vi "MergeFilesCreateFileHeader.vi"(4 "Error In":errorcluster, 7 "MergeFileConfig":T1) -> (0 "Error Out":errorcluster, 3 "TextFileHeader":string)   [LabVIEW 2017]
uses:
  DefDeType/MergeFileConfig.ctl
  DefDeType/WhichPath.ctl
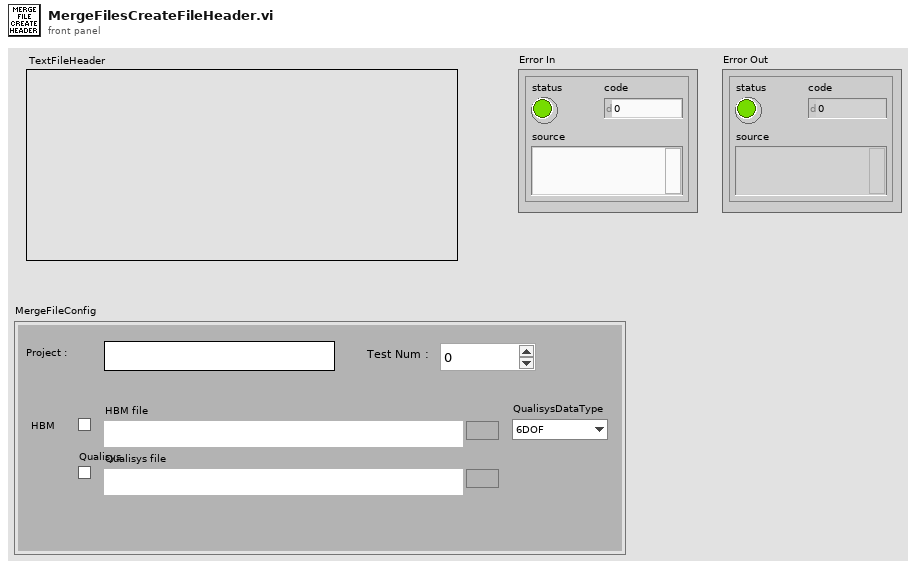
[diagram p1: front panel]
types:
  T1 = typedef "MergeFileConfig.ctl" = cluster{"Test Num : ":u32, "Project :":string, "Qualisys file":path, "HBM file":path, "QualisysDataType":enum16{"6DOF", "3DTracking", "6DOF + 3D"}, "Qualisys":bool, "HBM":bool}
  T2 = typedef "WhichPath.ctl" = enum16{"DossierProjet", "Config", "Meas", "MeasPCI", "MeasCRIO1", "MeasCRIO2", "MeasQualisys", "MeasHBM", "MeasTDMS", "Fig", "Res"}
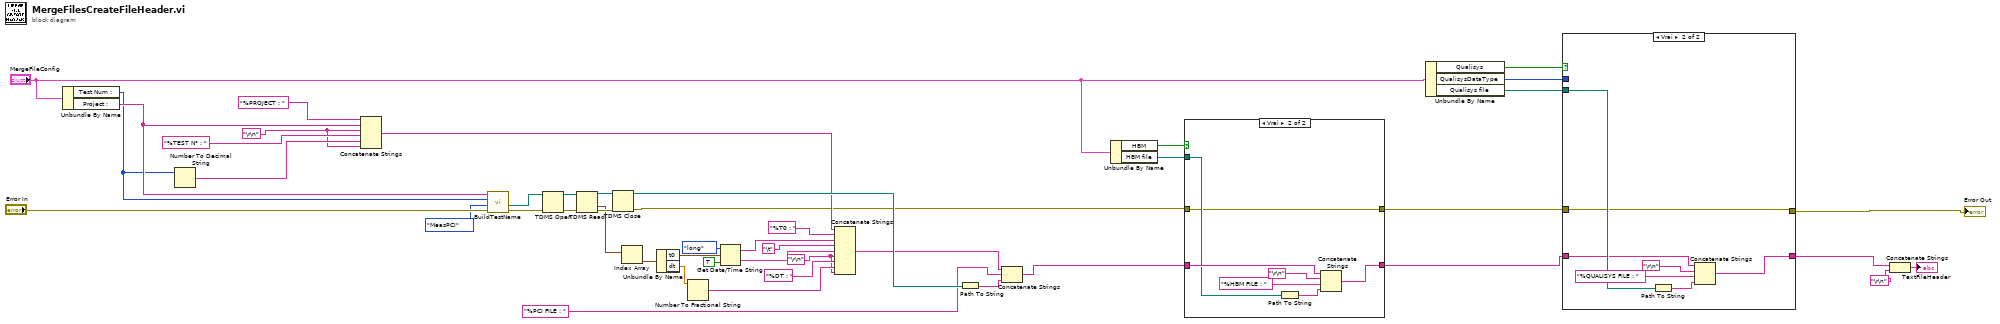
[diagram p0: block diagram]
diagram:
  w17 = "\r\n"
  w26 = "\r\n"
  n1 = Unbundle By Name("MergeFileConfig") -> ("Test Num :"=w15:u32, "Project :"=w16:string)
  n2 = Number To Decimal String(number=w15) -> (decimal integer string=w18:string)  [unwired: 1 in]
  n3 = Concatenate Strings("%PROJECT : " ("chaîne"), w16, w17, "%TEST N° : " ("chaîne"), w18, w17) -> (w14:string)
  n4 = call "BuildTestName.vi"("entrée d'erreur"="Error In", "WhichPath?"=WhichPath."MeasPCI", "NextTestNum"=w15, "NomProjet"=w16) -> ("sortie d'erreur"=w41:errorcluster, "cheminProchainFichier"=w42:path)  [unwired: 1 in, 2 out]
  n5 = TDMS Open(8:w41, 11:w42) -> (0:w44:errorcluster, 3:w43:refnum<k34>)  [unwired: 5 in]
  n6 = TDMS Read(0:w43, 11:w44) -> (4:w45:refnum<k34>, 10:w38:waveform(dbl)[], 15:w46:errorcluster)  [unwired: 6 in, 3 out]
  n7 = TDMS Close(8:w46, 11:w45) -> (0:w4:errorcluster, 3:w40:path)
  n8 = Index Array(array=w38) -> (element=w37:waveform(dbl))  [unwired: 1 in]
  n9 = Unbundle By Name(w37) -> ("t0"=w36:timestamp, "dt"=w29:dbl)
  n10 = Number To Fractional String(number=w29) -> (F-format string=w27:string)  [unwired: 3 in]
  n11 = Get Date/Time String(date format (0)=enum16{"short", "long", "abbreviated"}."long", seconds (now)=w36, want seconds? (F)=TRUE) -> (date string=w32:string, time string=w30:string)
  n12 = Concatenate Strings(w14, "%T0 : " ("Etat"), w32, "\t", w30, w26, "%DT : " ("Etat"), w27, w26) -> (w25:string)
  n13 = Path To String(path=w40) -> (string=w39:string)
  n14 = Concatenate Strings(w25, "%PCI FILE : " ("Etat"), w39) -> (w5:string)
  n15 = Unbundle By Name("MergeFileConfig") -> ("HBM"=w9:bool, "HBM file"=w8:path)
  n16 = case shown="Vrai" w9 {
    tunnel: w4 -> [w48 w49]
    tunnel: [w48 w49] -> w7
    tunnel: w8 -> [_ w50]
    tunnel: w5 -> [w47 w52]
    tunnel: [w47 w51] -> w6
    frame False {
    }
    frame True {
      n17 = Path To String(path=w50) -> (string=w54:string)
      n18 = Concatenate Strings(w52, "\r\n", "%HBM FILE : " ("Etat"), w54) -> (w51:string)
    }
  }
  n19 = Unbundle By Name("MergeFileConfig") -> ("Qualisys"=w23:bool, "QualisysDataType"=w22:enum16{"6DOF", "3DTracking", "6DOF + 3D"}, "Qualisys file"=w21:path)
  n20 = case shown="Vrai" w23 {
    tunnel: w22 -> [_ _]
    tunnel: w21 -> [_ w62]
    tunnel: w6 -> [w57 w60]
    tunnel: [w57 w59] -> w2
    tunnel: w7 -> [w56 w58]
    tunnel: [w56 w58] -> w3
    frame False {
    }
    frame True {
      n21 = Path To String(path=w62) -> (string=w63:string)
      n22 = Concatenate Strings(w60, "\r\n", "%QUALISYS FILE : " ("Etat"), w63) -> (w59:string)
    }
  }
  "Error Out" <- w3
  n23 = Concatenate Strings(w2, "\r\n") -> (→"TextFileHeader":string)
